vi "Obtaining Unknown Object References.vi"   [LabVIEW 2019]
doc: "This VI makes the labels of the control terminals in any target VI visible. Although this VI specifies a target VI, you can enter any target VI in the path to target VI control. Because this VI is intended to work for any target VI, the target VI is considered \"unknown.\" When a target VI is unknown until run time, the scripting VI can use the Traverse for GObjects VI to search for relevant objects.\n\nThe Detailed Help explains how this example illustrates a general procedure for obtaining references to objects in unknown target VIs."
uses:
  <vilib>/Utility/traverseref.llb/TRef TravTarget.ctl
  <vilib>/Utility/traverseref.llb/VI Scripting - Traverse.lvlib
panel:
  # "Select Help>>Show Context Help and move the cursor over the VI icon to display help for this VI.\n\nBefore you start: Open the Detailed Help for this example to display the Obtaining References to Objects in an Unknown Target VI Using VI Scripting topic in the  LabVIEW Help. That topic provides additional details about how this example illustrates the general procedure for obtaining references to objects in an unknown target VI.\n\nThis VI makes the labels of the control terminals in any target VI visible. Although this VI specifies a specific target VI, you can enter any target VI in the path to target VI control. Because this VI is intended to work for any target VI, the target VI is considered \"unknown.\" When a target VI is unknown until run time, the scripting VI can use the Traverse for GObjects VI to search for relevant objects.\n\nOpen the target VI to observe the effects of this scripting VI. The default target VI is located in labview\\examples\\Application Control\\VI Scripting\\Finding and Modifying Objects.\n\nTo run this VI more than once, close the target VI and do not save changes."
  # "Overview: Demonstrates the use of VI Scripting to programmatically manipulate a group of diagram objects that are all the same class.\nInstructions:\n1. Open Test - Obtaining Unknown Object References Target.vi.\n2. Run this VI. Observe that the labels of all control and indicator terminals on the block diagram become visible."
types:
  T1 = typedef "TRef TravTarget.ctl" = enum16{"FP", "BD", "Other"}
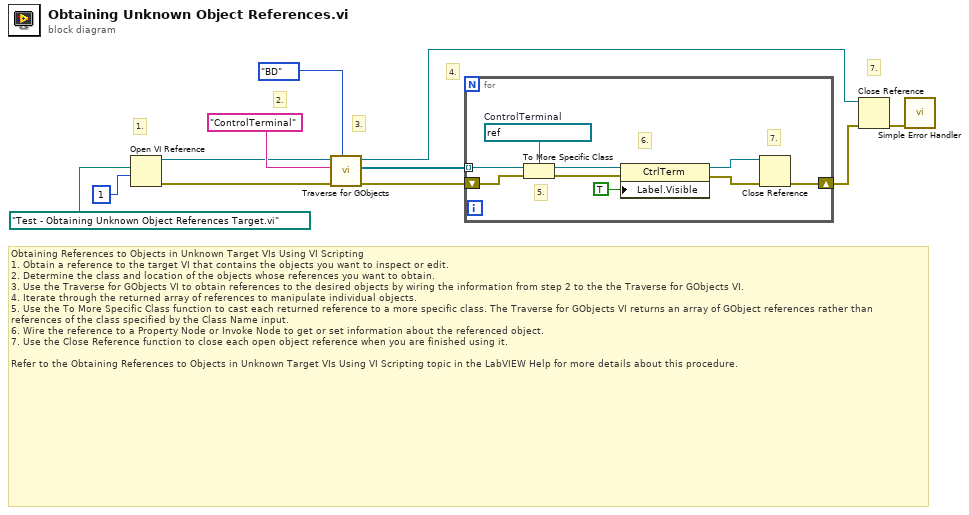
[diagram p0: block diagram]
diagram:
  # "7."
  # "4."
  # "3."
  # "2."
  # "1."
  # "Obtaining References to Objects in Unknown Target VIs Using VI Scripting\n1. Obtain a reference to the target VI that contains the objects you want to inspect or edit.\n2. Determine the class and location of the objects whose references you want to obtain.\n3. Use the Traverse for GObjects VI to obtain references to the desired objects by wiring the information from step 2 to the the Traverse for GObjects VI.\n4. Iterate through the returned array of references to manipulate individual objects.\n5. Use the To More Specific Class function to cast each returned reference to a more specific class. The Traverse for GObjects VI returns an array of GObject references rather than references of the class specified by the Class Name input.\n6. Wire the reference to a Property Node or Invoke Node to get or set information about the referenced object.\n7. Use the Close Reference function to close each open object reference when you are finished using it.\n\nRefer to the Obtaining References to Objects in Unknown Target VIs Using VI Scripting topic in the LabVIEW Help for more details about this procedure."
  n1 = Open VI Reference(vi path=path "Test - Obtaining Unknown Object References Target.vi" ("path to target VI"), options=1) -> (vi reference=w4:refnum<vi>, error out=w3:errorcluster)  [unwired: 4 in]
  n2 = call <vilib>:"Traverse for GObjects.vi"("Traverse Target"=TRef_TravTarget."BD", "error in (no error)"=w3, "Class Name"="ControlTerminal", "VI Refnum"=w4) -> ("error out"=w6:errorcluster, "References"=w9:refnum<vi>[], "dup VI Refnum"=w1:refnum<vi>)  [unwired: 4 in, 1 out]
  n3 = for {
    tunnel: w9 -> [w19] mode=indexing
    shift-right: [w15] -> w7
    shift-left: w6 -> [w12]
    w20 = refnum<vi> refnum  # ControlTerminal
    # "7."
    # "6."
    # "5."
    n4 = To More Specific Class(target class=w20, reference=w19, error in=w12) -> (specific class reference=w18:refnum<vi>, error out=w13:errorcluster)
    n5 = property on="Property Node" class="CtrlTerm"(reference=w18, error in=w13, "Label.Visible"=TRUE) -> (reference out=w17:refnum<vi>, error out=w14:errorcluster)
    n6 = Close Reference(reference=w17, error in (no error)=w14) -> (error out=w15:errorcluster)
  }
  n7 = Close Reference(reference=w1, error in (no error)=w7) -> (error out=w2:errorcluster)
  n8 = call <vilib>:"Simple Error Handler.vi"("error in (no error)"=w2) -> ()  [unwired: 4 in, 5 out]
